vi "Shutdown.vi"(8 "error in (no error)":errorcluster, 11 "Websocket Client in":refnum<class "Websocket Client.lvclass">) -> (0 "error out":errorcluster, 3 "Websocket Client out":refnum<class "Websocket Client.lvclass">)   [LabVIEW 2020, in "Stream-Websocket.lvlib" / "Websocket Client.lvclass"]
uses:
  Websocket Client.lvclass
  lv-stream/stream/Connection/Connection.lvclass
  lv-stream/stream/Connection/State.ctl
  Client Command.ctl
  Stream-Websocket.lvlib
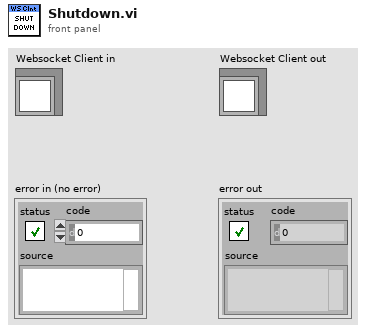
[diagram p1: front panel]
types:
  T1 = typedef "Stream-Websocket.lvlib/Client Command.ctl" = enum16{"Connect", "Close", "Shutdown", "Reconnect"}
  T2 = typedef "Stream.lvlib/Connection.lvclass/State.ctl" = enum16{"Closed", "Idle", "Connecting", "Connected", "Shutdown"}
  T3 = typedef "Stream-Websocket.lvlib/Websocket Client.lvclass/Ref Data.ctl" = cluster{"TCP Connection":refnum<k5>, "WS Stream":refnum<class "WebsocketStream.lvclass">, "Connection Loop":refnum<vi>, "Timeout ms":i32, "Server Connection":bool}
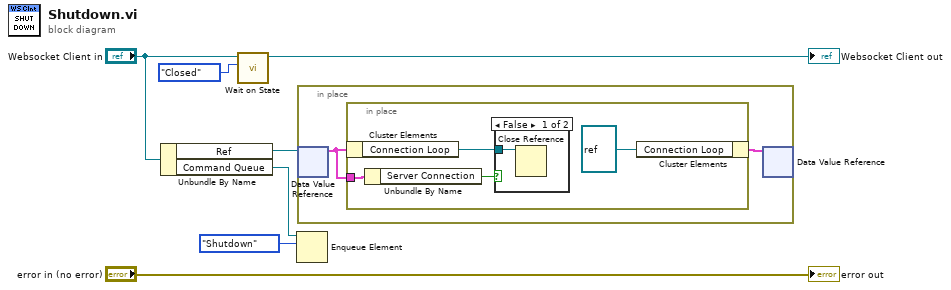
[diagram p0: block diagram]
diagram:
  n1 = Unbundle By Name("Websocket Client in") -> ("Ref"=w4:refnum<data-value>, "Command Queue"=w3:refnum<queue>)
  n2 = call "Wait on State.vi"("State"=State."Closed", "Connection in"="Websocket Client in") -> ("Connection out"=→"Websocket Client out":refnum<class "Websocket Client.lvclass">)  [unwired: 7 in, 2 out]
  n3 = Enqueue Element(queue=w3, element=Client_Command."Shutdown") -> ()  [unwired: 2 in, 3 out]
  n4 = in-place {
    n5 = in-place-dvr #1(w4) -> (w8:T3)  [unwired: 1 out]
    n6 = in-place {
      in-place-border: w8 -> [w13]
      n7 = in-place-cluster #2(w8) -> ("Connection Loop"=w11:refnum<vi>)
      n8 = Unbundle By Name(w13) -> ("Server Connection"=w12:bool)
      n9 = case shown="False" w12 {
        tunnel: w11 -> [w14 _]
        frame False {
          n10 = Close Reference(reference=w14) -> ()  [unwired: 1 in, 1 out]
        }
        frame True {
        }
      }
      n11 = in-place-cluster #2("Connection Loop"=refnum<vi> refnum) -> (w9:T3)
    }
    n12 = in-place-dvr #1(w9) -> ()  [unwired: 2 out]
  }
  "error out" <- "error in (no error)"
